vi "Read Y.vi"(2 "error in (no error)":errorcluster, 3 "Sensor.lvclass":refnum<class "Sensor.lvclass">) -> (0 "error out":errorcluster, 1 "Y":dbl)   [LabVIEW 2015, in "Sensor.lvclass"]
uses:
  Sensor.lvclass
  Sensor.lvclass/Sensor.ctl
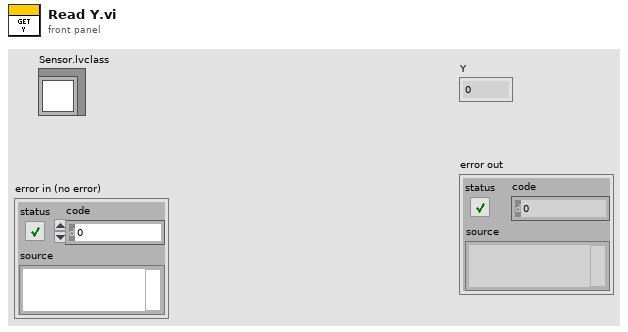
[diagram p1: front panel]
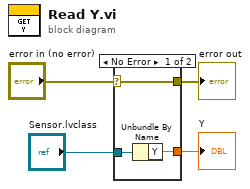
[diagram p0: block diagram]
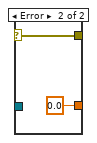
[diagram p2: hidden frame]
diagram:
  n1 = case shown="No Error" "error in (no error)" {
    selector: "error in (no error)" -> [w7 w9]
    tunnel: [w7 w9] -> w3
    tunnel: "Sensor.lvclass" -> [w6 _]
    tunnel: [w5 0.0] -> w1
    frame No Error {
      n2 = Unbundle By Name(w6) -> ("Y"=w5:dbl)
    }
    frame Error {
    }
  }
  "Y" <- w1
  "error out" <- w3
